vi "GetFinalFrameBit.vi"(9 "Byte Packet":u8) -> (0 "Final Frame Bit":bool, 2 "Byte Packet out":u8)   [LabVIEW 2017, in "LV WebSockets.lvlib"]
uses:
  LV WebSockets.lvlib
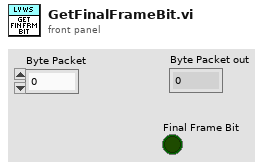
[diagram p1: front panel]
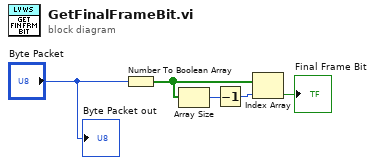
[diagram p0: block diagram]
diagram:
  n1 = Number To Boolean Array(number="Byte Packet") -> (Boolean array=w3:bool[])
  n2 = Array Size(array=w3) -> (size(s)=w5:i32)
  n3 = Decrement(x=w5) -> (x-1=w4:i32)
  n4 = Index Array(array=w3, index=w4) -> (element=→"Final Frame Bit":bool)
  "Byte Packet out" <- "Byte Packet"
